vi "uptospeed.vi"(7 "Description":string, 8 "Command Info In":T1, 10 "on of":dbl, 11 "Setpoint":dbl) -> (0 "Command Info Out":T1)   [LabVIEW 2015]
uses:
  <vilib>/Rock Robotics/WPI/Framework/Command Status Info.ctl
  <vilib>/Rock Robotics/WPI/Framework/Completion Status.ctl
  <vilib>/Rock Robotics/WPI/Framework/Completion Notifier.ctl
  Implementation/shooter Setpoints.ctl
  Implementation/shooter Operations.ctl
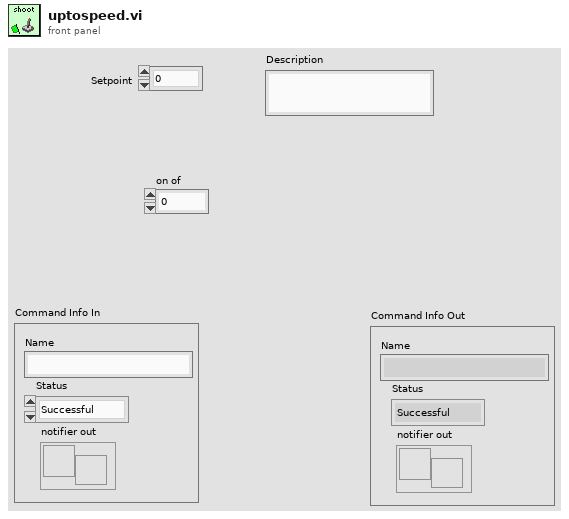
[diagram p1: front panel]
types:
  T1 = typedef "Command Status Info.ctl" = cluster{"Name":string, "Status":T2, "notifier out":T3}
  T2 = typedef "Completion Status.ctl" = enum16{"Successful", "Aborted", "Incomplete"}
  T3 = typedef "Completion Notifier.ctl" = refnum<notifier>
  T4 = typedef "shooter Setpoints.ctl" = cluster{"Operation":T5, "Setpoint":dbl, "Duration":dbl, "PID Angle Setpoint":dbl, "cowl on/off":dbl}
  T5 = typedef "shooter Operations.ctl" = enum16{"Reserve", "Read Current", "Immediate", "UpToSpeed", "MoveToAngle"}
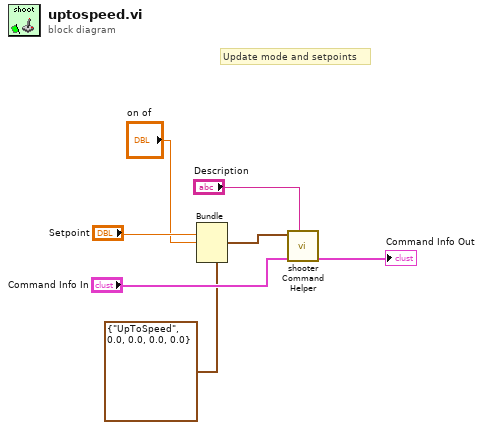
[diagram p0: block diagram]
diagram:
  # "Update mode and setpoints"
  n1 = Bundle(cluster=T4 {"Operation"=enum."UpToSpeed", "Setpoint"=0.0, "Duration"=0.0, "PID Angle Setpoint"=0.0, "cowl on/off"=0.0} ("SubSystem Data"), "Setpoint"="Setpoint", "Duration"="on of") -> (w2:T4)  [unwired: 3 in]
  n2 = call "shooter Command Helper.vi"("Description"="Description", "Command Info In"="Command Info In", "SubSystem Data"=w2) -> ("Command Info Out"=→"Command Info Out":T1)  [unwired: 7 in, 1 out]
